vi "Is Concrete Class.vi"(0 "SA 26GHz Path Group in":refnum<class "SA 26GHz Path Group.lvclass">, 11 "error in":errorcluster) -> (4 "SA 26GHz Path Group out":refnum<class "SA 26GHz Path Group.lvclass">, 6 "Is Concrete Class?":bool, 15 "error out":errorcluster)   [LabVIEW 2023, in "RFFixtureCharact.PXI.lvlib" / "SA 26GHz Path Group.lvclass"]
uses:
  SA 26GHz Path Group.lvclass
  SA 26GHz Path Group.lvclass/SA 26GHz Path Group.ctl
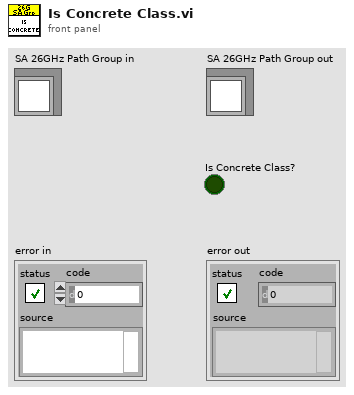
[diagram p1: front panel]
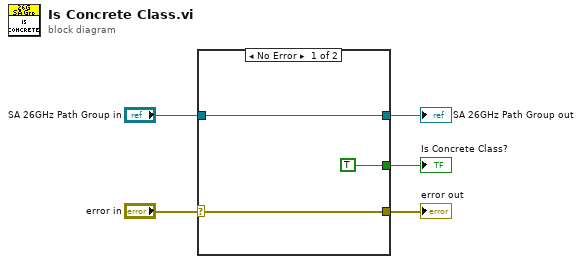
[diagram p0: block diagram]
diagram:
  n1 = case shown="No Error" "error in" {
    selector: "error in" -> [w7 w9]
    tunnel: [TRUE ("Is Concrete Class?") _] -> w3
    tunnel: [w7 w9] -> w2
    tunnel: [w6 w10] -> w4
    tunnel: "SA 26GHz Path Group in" -> [w6 w10]
    frame No Error {
    }
    frame Error {
    }
  }
  "error out" <- w2
  "SA 26GHz Path Group out" <- w4
  "Is Concrete Class?" <- w3
